vi "CICP I64 Tag.vi"() -> (3 "CIF_CIPC_Chn_I64.lvclass":refnum<class "CIF_CIPC_Chn_I64.lvclass">)   [LabVIEW 2021, in "CIF_CIPC_Chn_I64.lvclass"]
uses:
  CIF_CIPC_Chn_I64.lvclass
  CIF_CIPC_Chn_I64.lvclass/CIF_CIPC_Chn_I64.ctl
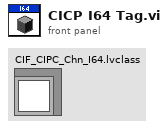
[diagram p1: front panel]
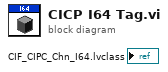
[diagram p0: block diagram]
diagram:
